vi "LVClass_WavefrontCorrectorSet ReadFile WavefrontCorrectorSetup.vi"(0 "WavefrontCorrectorSet in":refnum<class "WavefrontCorrectorSet.lvclass">, 11 "error in (no error)":errorcluster) -> (4 "WavefrontCorrectorSet out":refnum<class "WavefrontCorrectorSet.lvclass">, 15 "error out":errorcluster)   [LabVIEW 2020, in "WavefrontCorrectorSet.lvclass"]
uses:
  WavefrontCorrectorSet.lvclass
  CameraParametersSetup.ctl
  CameraParameters_Type.ctl
  Wavefront Corrector states.ctl
  Wavefront Corrector states - ONE.ctl
  WavefrontCorrectorSet.lvclass/WavefrontCorrectorSet.ctl
  Read From XML File(string).vi
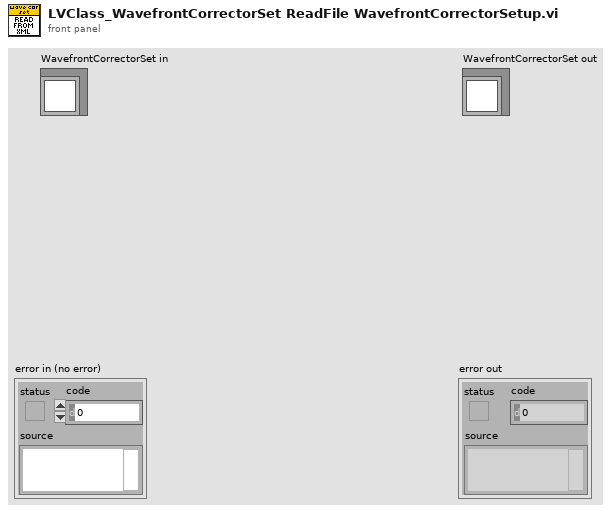
[diagram p1: front panel]
types:
  T1 = typedef "CameraParametersSetup.ctl" = cluster{"Name":string, "Type":T2, "Value":dbl, "BooleanValue":bool, "StringValue":string}
  T2 = typedef "CameraParameters_Type.ctl" = enum16{"Integer", "Real", "String", "Boolean"}
  T3 = typedef "Wavefront Corrector states.ctl" = cluster{"Sleep after command apply_ms":i32, "Wavefront Corrector State":T4[], "WavefrontCorrectorOffsetState":sgl[]}
  T4 = typedef "Wavefront Corrector states - ONE.ctl" = cluster{"Max":sgl, "Min":sgl, "Validity":enum16{"valid", "fixed", "invalid"}, "Fixed_Position":sgl}
  T5 = cluster{"AllWavefrontCorrectorParameters":T1[], "WavefrontCorrectorPreferences":T3}
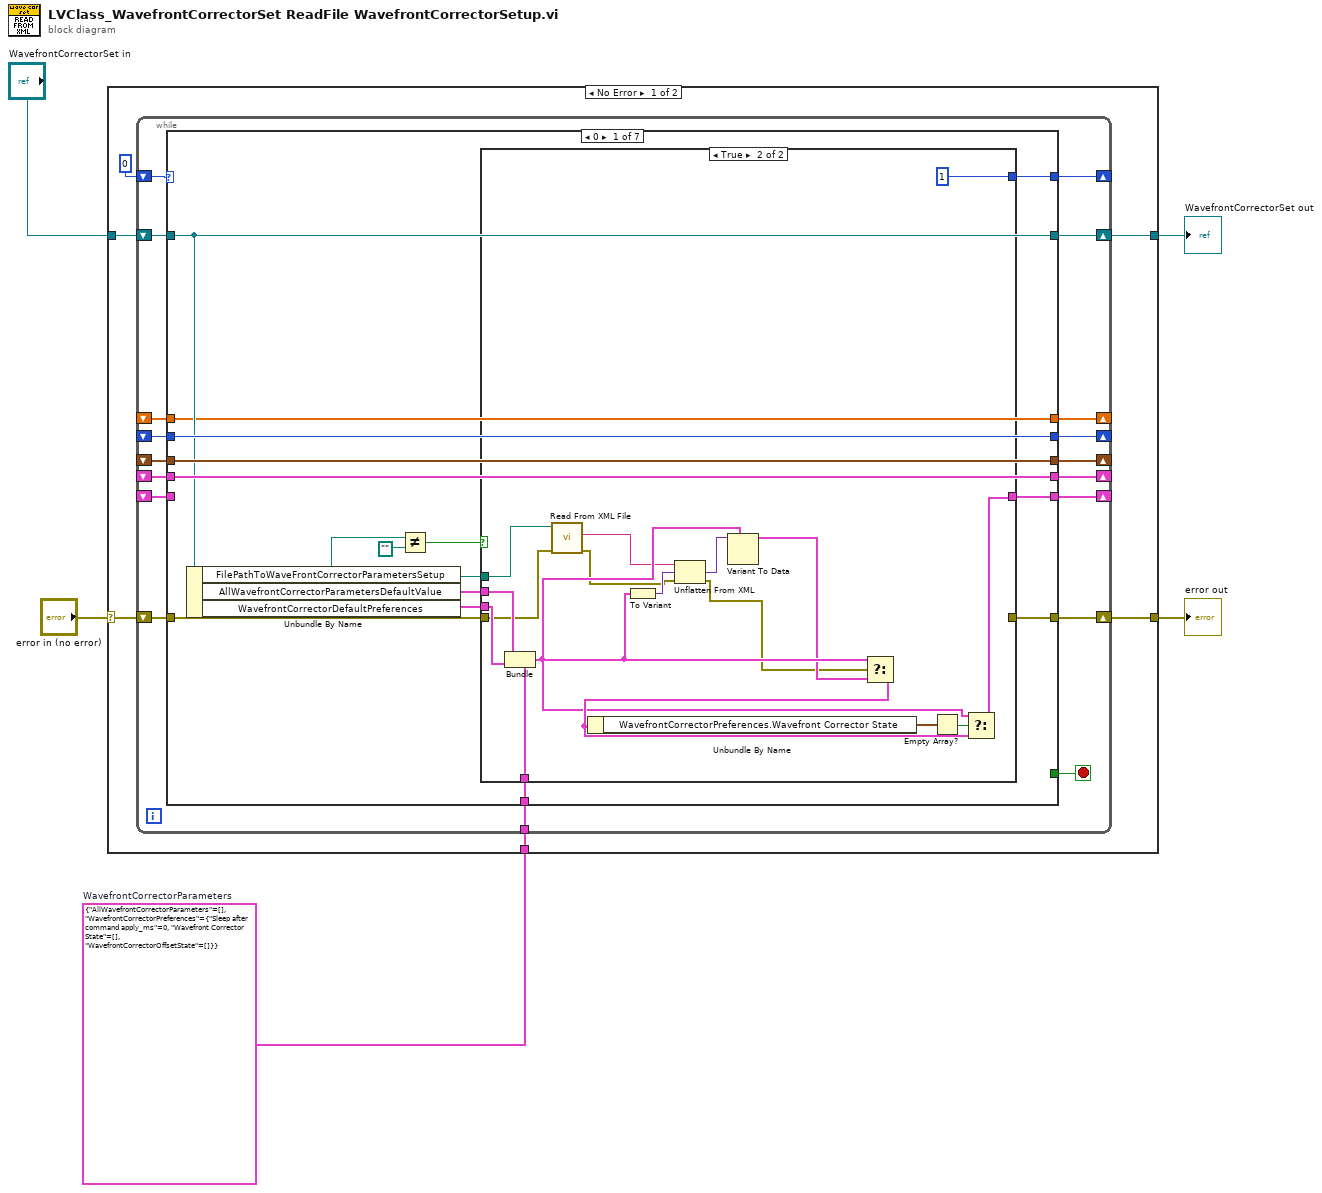
[diagram p0: block diagram]
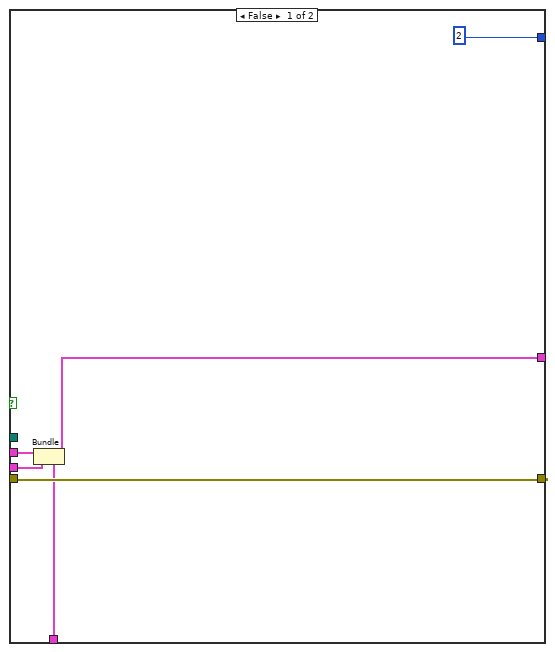
[diagram p2: hidden frame]
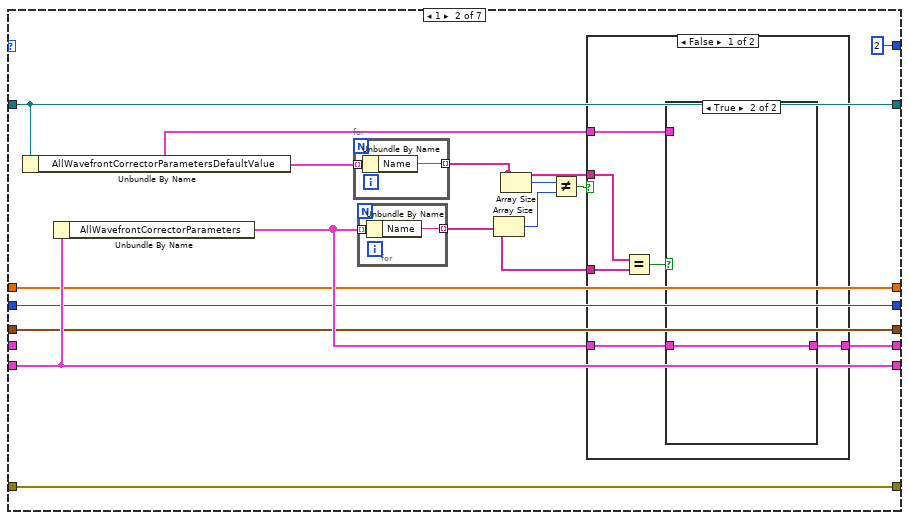
[diagram p3: hidden frame]
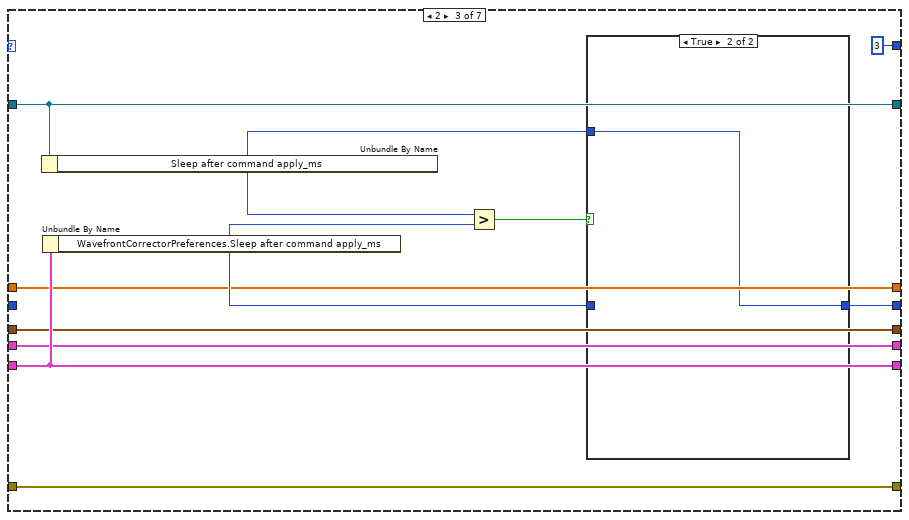
[diagram p6: hidden frame]
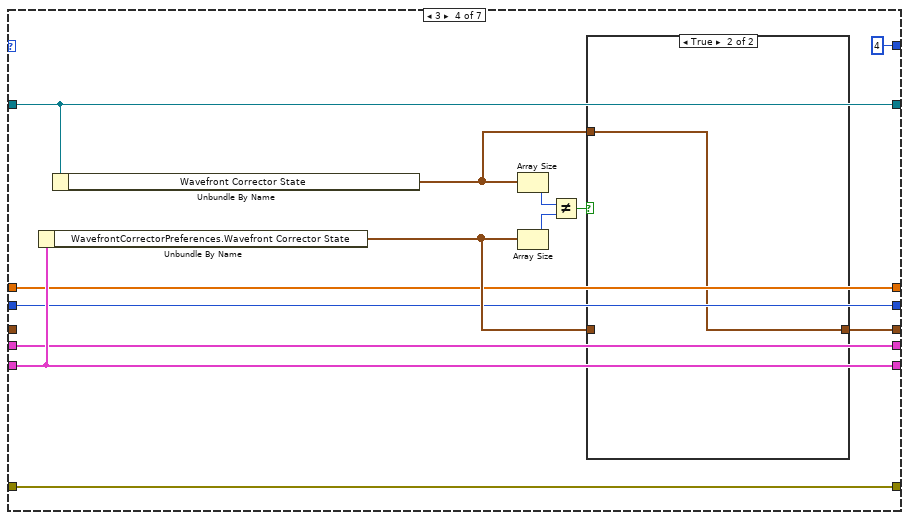
[diagram p8: hidden frame]
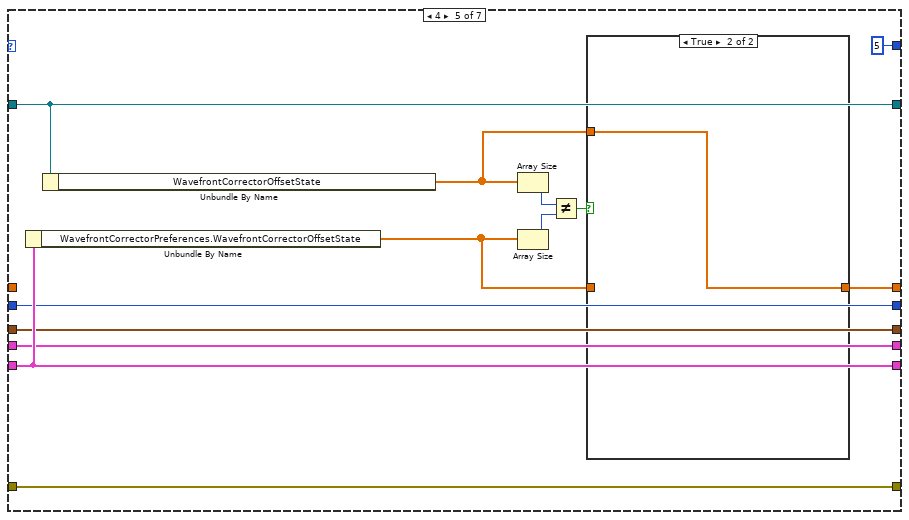
[diagram p10: hidden frame]
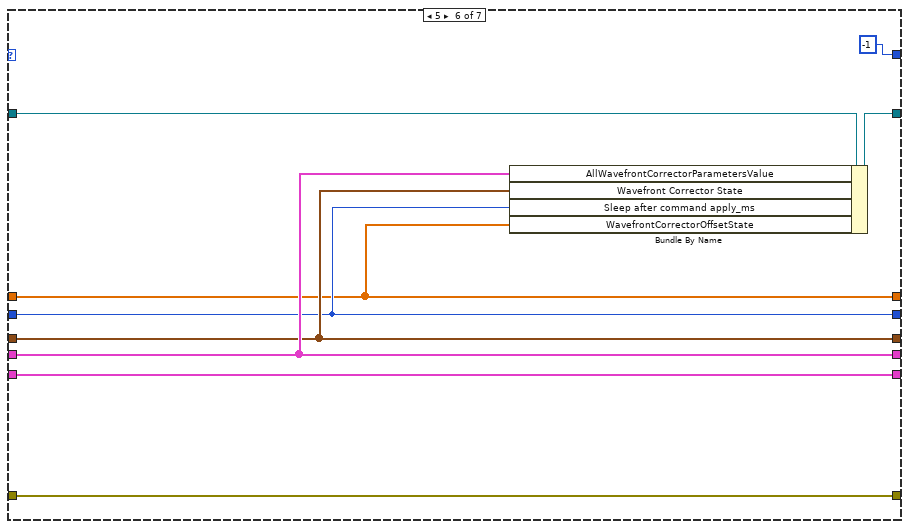
[diagram p12: hidden frame]
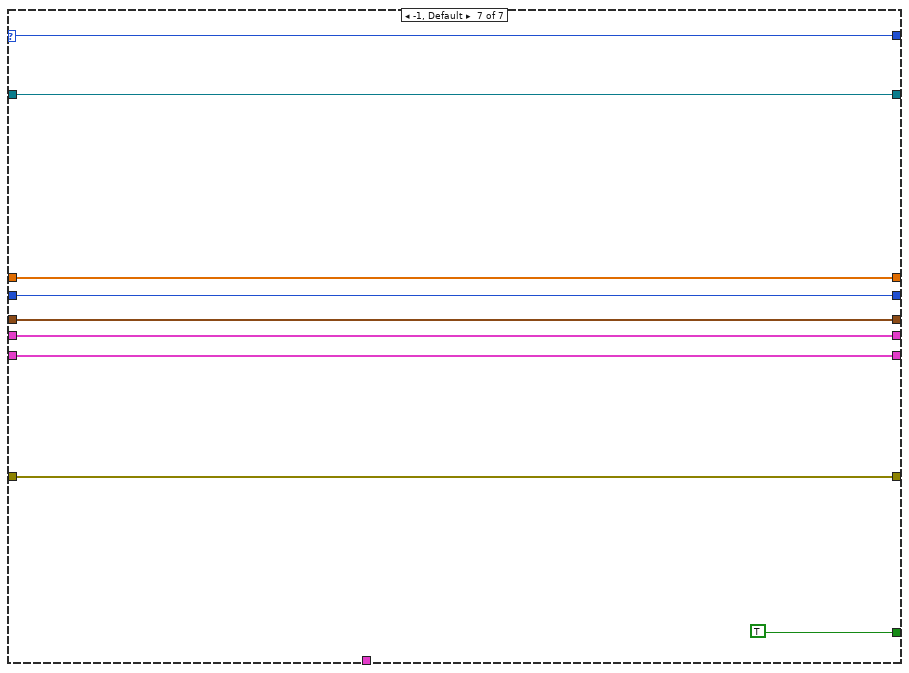
[diagram p13: hidden frame]
diagram:
  w1 = T5 {"AllWavefrontCorrectorParameters"=[], "WavefrontCorrectorPreferences"={"Sleep after command apply_ms"=0, "Wavefront Corrector State"=[], "WavefrontCorrectorOffsetState"=[]}}  # WavefrontCorrectorParameters
  n1 = case shown="No Error" "error in (no error)" {
    selector: "error in (no error)" -> [w10 w158]
    tunnel: [w11 w158] -> w4
    tunnel: "WavefrontCorrectorSet in" -> [w8 w157]
    tunnel: [w7 w157] -> w2
    tunnel: w1 -> [w6 _]
    frame No Error {
      n2 = while {
        shift-right: [w27] -> _
        shift-left: _ -> [w23]
        shift-right: [w21] -> _
        shift-left: 0 -> [w25]
        shift-right: [w22] -> w7
        shift-left: w8 -> [w26]
        shift-right: [w29] -> w11
        shift-left: w10 -> [w28]
        tunnel: w6 -> [w20]
        shift-right: [w17] -> _
        shift-left: _ -> [w16]
        shift-right: [w19] -> _
        shift-left: _ -> [w18]
        shift-right: [w15] -> _
        shift-left: _ -> [w14]
        shift-right: [w13] -> _
        shift-left: _ -> [w12]
        stop <- w24 stop-if-true
        n3 = case shown="0" w25 {
          selector: w25 -> [_ _ _ _ _ _ w152]
          tunnel: [w44 w74 w104 w116 w131 w144 w155] -> w29
          tunnel: w28 -> [w43 w74 w104 w116 w131 w144 w155]
          tunnel: [w39 w72 w103 w115 w130 w143 w154] -> w27
          tunnel: w26 -> [w31 w81 w105 w120 w135 w147 w153]
          tunnel: [_ _ _ _ _ _ TRUE] -> w24
          tunnel: w23 -> [_ w72 w103 w115 w130 w143 w154]
          tunnel: [w31 w81 w105 w120 w135 w146 w153] -> w22
          tunnel: [w37 2 3 4 5 -1 w152] -> w21
          tunnel: w20 -> [w36 _ _ _ _ _ _]
          tunnel: [w34 w73 w100 w112 w127 w142 w150] -> w19
          tunnel: w18 -> [w34 _ w100 w112 w127 w142 w150]
          tunnel: [w33 w70 w102 w111 w125 w141 w151] -> w17
          tunnel: w16 -> [w33 w70 w102 _ w125 w141 w151]
          tunnel: [w32 w69 w101 w110 w126 w140 w149] -> w15
          tunnel: w14 -> [w32 w69 _ w110 w126 w140 w149]
          tunnel: [w30 w68 w96 w109 w124 w139 w148] -> w13
          tunnel: w12 -> [w30 w68 w96 w109 _ w139 w148]
          frame 0 {
            n4 = Unbundle By Name(w31) -> ("FilePathToWaveFrontCorrectorParametersSetup"=w41:path, "AllWavefrontCorrectorParametersDefaultValue"=w38:T1[], "WavefrontCorrectorDefaultPreferences"=w35:T3)
            n5 = Not Equal?(x=w41, y=path "") -> (x != y?=w40:bool)
            n6 = case shown="True" w40 {
              tunnel: w41 -> [_ w56]
              tunnel: [w50 _] -> w44
              tunnel: w43 -> [w50 w57]
              tunnel: [w46 w66] -> w39
              tunnel: w38 -> [w47 w62]
              tunnel: [2 1] -> w37
              tunnel: w36 -> [w45 w64]
              tunnel: w35 -> [w48 w63]
              frame False {
                n7 = Bundle(cluster=w45, "AllWavefrontCorrectorParameters"=w47, "WavefrontCorrectorPreferences"=w48) -> (w46:T5)
              }
              frame True {
                n8 = Bundle(cluster=w64, "AllWavefrontCorrectorParameters"=w62, "WavefrontCorrectorPreferences"=w63) -> (w59:T5)
                n9 = call-poly "Read From XML File.vi"("error in (no error)"=w57, "XML File Path"=w56) -> ("error out"=w52:errorcluster, "XML Elements"=w55:string)  [unwired: 7 in, 1 out]
                n10 = To Variant(anything=w59) -> (Variant=w54:variant)
                n11 = Unflatten From XML(xml string=w55, type=w54, error in (no error)=w52) -> (value=w53:variant, error out=w51:errorcluster)
                n12 = Variant To Data(type=w59, Variant=w53) -> (data=w58:T5)  [unwired: 1 in, 1 out]
                n13 = Select(t=w59, s=w51, f=w58) -> (s? t:f=w60:T5)
                n14 = Unbundle By Name(w60) -> ("WavefrontCorrectorPreferences.Wavefront Corrector State"=w61:T4[])
                n15 = Empty Array?(array=w61) -> (empty?=w67:bool)
                n16 = Select(t=w59, s=w67, f=w60) -> (s? t:f=w66:T5)
              }
            }
          }
          frame 1 {
            n17 = Unbundle By Name(w81) -> ("AllWavefrontCorrectorParametersDefaultValue"=w77:T1[])
            n18 = Unbundle By Name(w72) -> ("AllWavefrontCorrectorParameters"=w71:T1[])
            n19 = for {
              tunnel: w77 -> [w93] mode=indexing
              tunnel: [w92] -> w76 mode=indexing
              n20 = Unbundle By Name(w93) -> ("Name"=w92:string)
            }
            n21 = for {
              tunnel: w71 -> [w95] mode=indexing
              tunnel: [w94] -> w75 mode=indexing
              n22 = Unbundle By Name(w95) -> ("Name"=w94:string)
            }
            n23 = Array Size(array=w75) -> (size(s)=w79:i32)
            n24 = Array Size(array=w76) -> (size(s)=w80:i32)
            n25 = Not Equal?(x=w80, y=w79) -> (x != y?=w78:bool)
            n26 = case shown="False" w78 {
              tunnel: w77 -> [w83 w91]
              tunnel: [w85 w91] -> w73
              tunnel: w76 -> [w88 _]
              tunnel: w75 -> [w87 _]
              tunnel: w71 -> [w84 _]
              frame False {
                n27 = Equal?(x=w88, y=w87) -> (x = y?=w86:bool)
                n28 = case shown="True" w86 {
                  tunnel: [w89 w90] -> w85
                  tunnel: w84 -> [_ w90]
                  tunnel: w83 -> [w89 _]
                  frame False {
                  }
                  frame True {
                  }
                }
              }
              frame True {
              }
            }
          }
          frame 2 {
            n29 = Unbundle By Name(w105) -> ("Sleep after command apply_ms"=w99:i32)
            n30 = Unbundle By Name(w103) -> ("WavefrontCorrectorPreferences.Sleep after command apply_ms"=w98:i32)
            n31 = Greater?(x=w99, y=w98) -> (0:w97:bool)
            n32 = case shown="True" w97 {
              tunnel: w99 -> [_ w108]
              tunnel: w98 -> [w107 _]
              tunnel: [w107 w108] -> w101
              frame False {
              }
              frame True {
              }
            }
          }
          frame 3 {
            n33 = Unbundle By Name(w115) -> ("WavefrontCorrectorPreferences.Wavefront Corrector State"=w113:T4[])
            n34 = Unbundle By Name(w120) -> ("Wavefront Corrector State"=w114:T4[])
            n35 = Array Size(array=w114) -> (size(s)=w119:i32)
            n36 = Array Size(array=w113) -> (size(s)=w118:i32)
            n37 = Not Equal?(x=w119, y=w118) -> (x != y?=w117:bool)
            n38 = case shown="True" w117 {
              tunnel: w114 -> [_ w123]
              tunnel: [w122 w123] -> w111
              tunnel: w113 -> [w122 _]
              frame False {
              }
              frame True {
              }
            }
          }
          frame 4 {
            n39 = Unbundle By Name(w130) -> ("WavefrontCorrectorPreferences.WavefrontCorrectorOffsetState"=w128:sgl[])
            n40 = Unbundle By Name(w135) -> ("WavefrontCorrectorOffsetState"=w129:sgl[])
            n41 = Array Size(array=w129) -> (size(s)=w134:i32)
            n42 = Array Size(array=w128) -> (size(s)=w133:i32)
            n43 = Not Equal?(x=w134, y=w133) -> (x != y?=w132:bool)
            n44 = case shown="True" w132 {
              tunnel: w129 -> [_ w138]
              tunnel: w128 -> [w137 _]
              tunnel: [w137 w138] -> w124
              frame False {
              }
              frame True {
              }
            }
          }
          frame 5 {
            n45 = Bundle By Name(cluster=w147, "AllWavefrontCorrectorParametersValue"=w142, "Wavefront Corrector State"=w141, "Sleep after command apply_ms"=w140, "WavefrontCorrectorOffsetState"=w139) -> (w146:refnum<class "WavefrontCorrectorSet.lvclass">)
          }
          frame -1, Default {
          }
        }
      }
    }
    frame Error {
    }
  }
  "error out" <- w4
  "WavefrontCorrectorSet out" <- w2
